vi "Generate Simulated Data.vi"(6 "Acquisition":refnum<queue>, 8 "error in (no error)":errorcluster, 10 "Longueur d'onde":dbl, 11 "Loop Count":dbl) -> (0 "error out":errorcluster, 2 "Data Out":variant[](array[variant]), 3 "Disconnected":bool=TRUE)   [LabVIEW 2018, in "Acquisition.lvlib"]
doc: "Generates sample waveforms according to the signal type in the HW Config input."
uses:
  Acquisition.lvlib
  <vilib>/Analysis/NI_AALBase.lvlib
  GlobalVariable/GlobalPowerByTime.vi
  GlobalVariable/Globalt0.vi
  support/Message Queue/Message Queue.lvlib
  <vilib>/gmath/NI_Gmath.lvlib
  GlobalVariable/GlobalSet0.vi
  <vilib>/Analysis/NI_AALPro.lvlib
  GlobalVariable/GlobalPosXbyTime.vi
  GlobalVariable/GlobalPosYbyTime.vi
  GlobalVariable/GlobalProfileByTime.vi
  GlobalVariable/GlobalTimeStep.vi
  GlobalVariable/GlobalTensionByTime.vi
  GlobalVariable/GlobalTemperatureByTime.vi
  support/Message Queue/Enqueue Message (Single).vi
  <vilib>/gmath/interp.llb/Create Mesh Grid (2D) (x,y arrays).vi
  <vilib>/Analysis/2dsp.llb/2D Convolution (DBL).vi
  <vilib>/Analysis/baseanly.llb/Mean (DBL).vi
  <vilib>/DAQmx/create/channels.llb/DAQmx Create Channel (DO-Digital Output).vi
  <resource>/objmgr/daqmx.rc
  <vilib>/DAQmx/write.llb/DAQmx Write (Digital 1D Bool NChan 1Samp 1Line).vi
  <vilib>/DAQmx/create/channels.llb/DAQmx Create Channel (AI-Voltage-Basic).vi
  <vilib>/DAQmx/configure/timing.llb/DAQmx Timing (Sample Clock).vi
  <vilib>/DAQmx/read.llb/DAQmx Read (Analog 1D Wfm NChan NSamp).vi
  support/Message Queue/Message Cluster.ctl
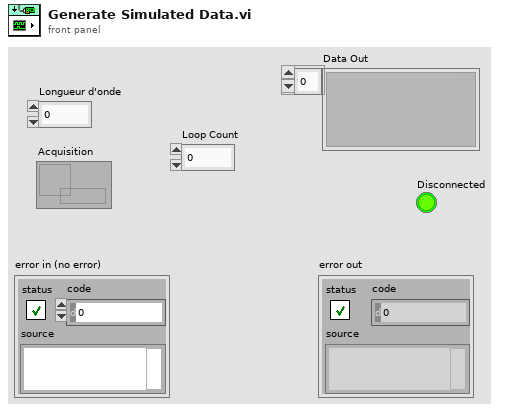
[diagram p1: front panel]
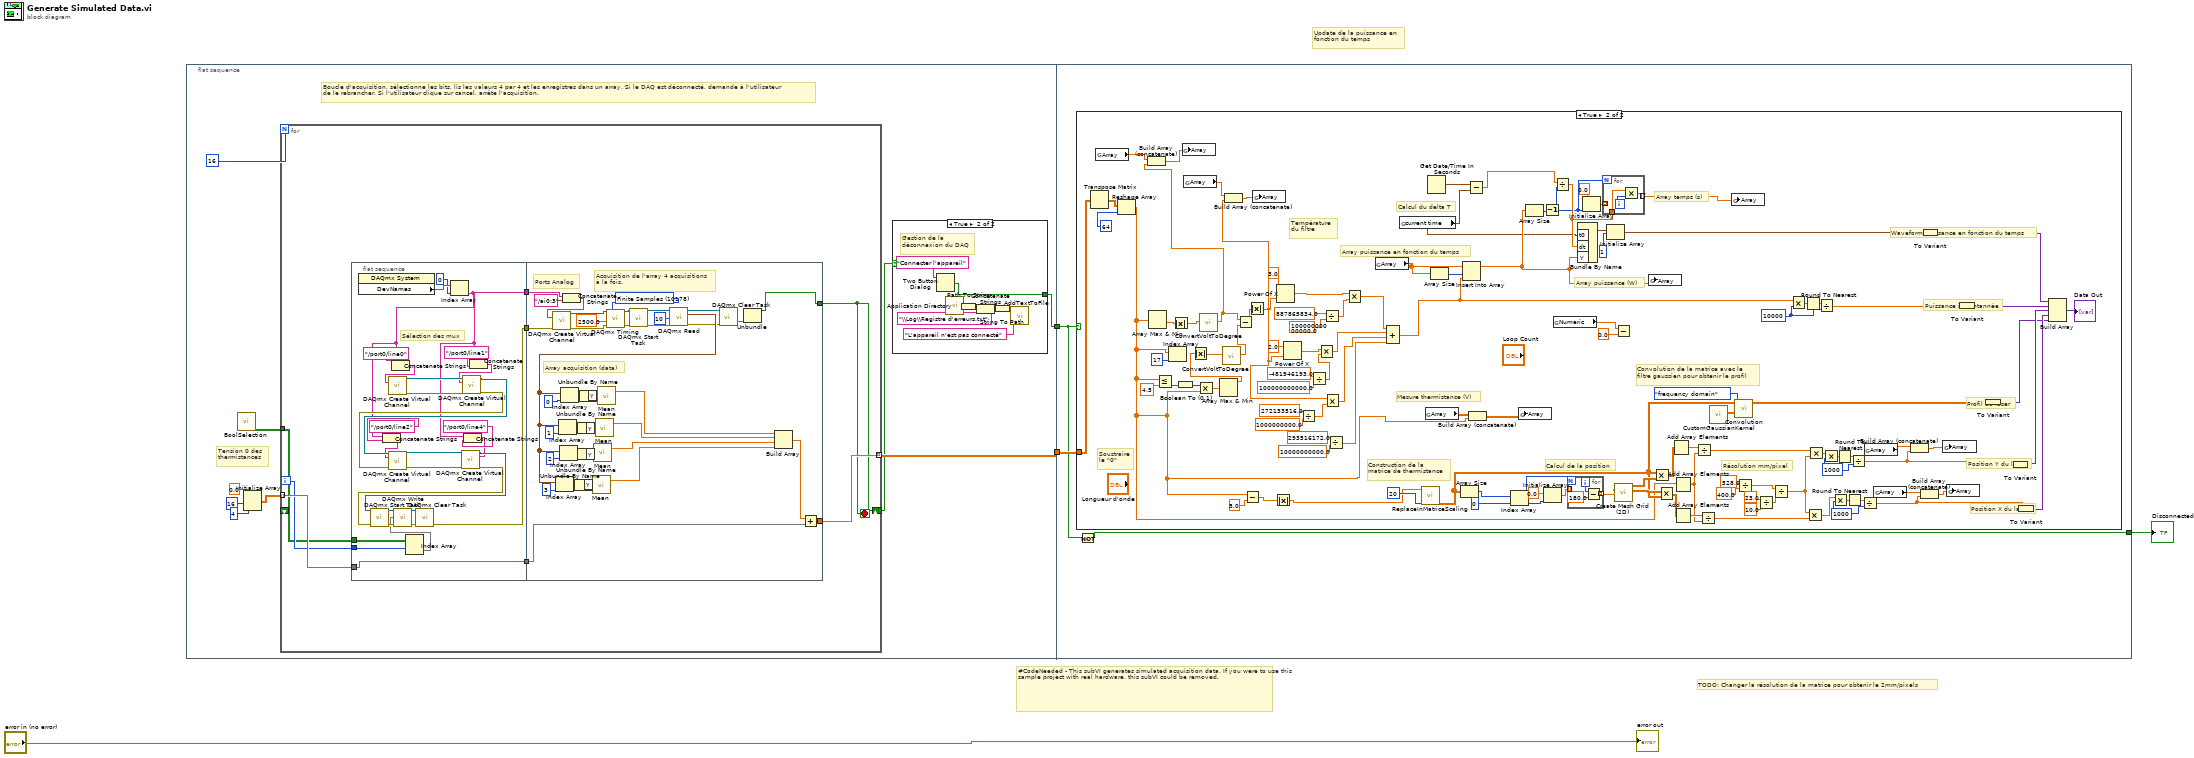
[diagram p0: block diagram]
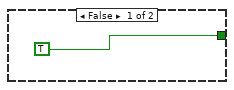
[diagram p2: hidden frame]
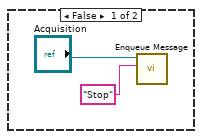
[diagram p3: hidden frame]
diagram:
  # "TODO: Changer la résolution de la matrice pour obtenir le 2mm/pixels"
  # "Update de la puissance en\nfonction du temps"
  # "#CodeNeeded - This subVI generates simulated acquisition data. If you were to use this sample project with real hardware, this subVI could be removed."
  n1 = flat-sequence {
    tunnel: [w11] -> w3
    tunnel: [w10] -> w2
    tunnel: w3 -> [w98]
    tunnel: w2 -> [w97]
    tunnel: [w96] -> w1
    frame #0 {
      # "Boucle d'acquisition, sélectionne les bits, lis les valeurs 4 par 4 et les enregistres dans un array. Si le DAQ est déconnecté, demande à l'utilisateur \nde le rebrancher. Si l'utilisateur clique sur cancel, arrête l'acquisition."
      # "Tension 0 des \nthermistances"
      n2 = call "BoolSelection.vi"() -> ("BoolSelection"=w12:bool[][])  [unwired: 11 in]
      n3 = Initialize Array(0.0 ("element"), 16 ("dimension size"), 4 ("dimension size")) -> (w6:dbl[][])
      n4 = for {
        N: 16 -> [_]
        tunnel: w12 -> [w25]
        tunnel: w6 -> [w30] mode=indexing
        tunnel: [w24] -> w11 mode=indexing
        shift-right: [w23] -> w5
        shift-left: _ -> [_]
        i -> [w26]
        stop <- w23 stop-if-true
        n5 = flat-sequence {
          tunnel: w26 -> [w44]
          tunnel: [w55] -> w29
          tunnel: w25 -> [w43]
          tunnel: [w31] -> w28
          tunnel: [w32] -> w27
          tunnel: w30 -> [w31]
          tunnel: w29 -> [w87]
          tunnel: w28 -> [w67]
          tunnel: [w69] -> w24
          tunnel: w27 -> [w64]
          tunnel: [w59] -> w23
          frame #0 {
            # "Sélection des mux"
            n6 = property class="DAQmx System"() -> ("DevNames"=w42:tag[])  [unwired: 2 in, 2 out]
            n7 = Index Array(array=w43, index (row)=w44) -> (element=w56:bool[])  [unwired: 1 in]
            n8 = Index Array(array=w42, index=0) -> (element=w32:tag)
            n9 = Concatenate Strings(w32, "/port0/line2" ("string")) -> (w35:string)
            n10 = Concatenate Strings(w32, "/port0/line0" ("string")) -> (w40:string)
            n11 = call-poly <vilib>:"DAQmx Create Virtual Channel.vi"("lines"=w40) -> ("task out"=w51:refnum<k21>, "error out"=w52:errorcluster)  [unwired: 13 in]
            n12 = Concatenate Strings(w32, "/port0/line4" ("string")) -> (w33:string)
            n13 = Concatenate Strings(w32, "/port0/line1" ("string")) -> (w37:string)
            n14 = call-poly <vilib>:"DAQmx Create Virtual Channel.vi"("task in"=w51, "lines"=w37, "error in"=w52) -> ("task out"=w50:refnum<k21>, "error out"=w49:errorcluster)  [unwired: 11 in]
            n15 = call-poly <vilib>:"DAQmx Create Virtual Channel.vi"("task in"=w50, "lines"=w35, "error in"=w49) -> ("task out"=w47:refnum<k21>, "error out"=w48:errorcluster)  [unwired: 11 in]
            n16 = call-poly <vilib>:"DAQmx Create Virtual Channel.vi"("task in"=w47, "lines"=w33, "error in"=w48) -> ("task out"=w46:refnum<k21>, "error out"=w45:errorcluster)  [unwired: 11 in]
            n17 = call <vilib>:"DAQmx Start Task.vi"("task/channels in"=w46, "error in"=w45) -> ("task out"=w57:refnum<k21>, "error out"=w58:errorcluster)  [unwired: 12 in]
            n18 = call-poly <vilib>:"DAQmx Write.vi"("task/channels in"=w57, "data"=w56, "error in"=w58) -> ("task out"=w54:refnum<k21>, "error out"=w53:errorcluster)  [unwired: 10 in, 1 out]
            n19 = call <vilib>:"DAQmx Clear Task.vi"("task in"=w54, "error in"=w53) -> ("error out"=w55:errorcluster)  [unwired: 13 in]
          }
          frame #1 {
            w89 = 10178 items=["Finite Samples"=10178, "Continuous Samples"=10123, "Hardware Timed Single Point"=12522] ("sample mode")
            # "Ports Analog"
            # "Array acquisition (data)"
            # "Acquisition de l'array 4 acquisitions\nà la fois."
            n20 = Concatenate Strings(w64, "/ai0:3" ("string")) -> (w65:string)
            n21 = call-poly <vilib>:"DAQmx Create Virtual Channel.vi"("physical channels"=w65, "error in"=w87) -> ("task out"=w94:refnum<k21>, "error out"=w93:errorcluster)  [unwired: 12 in]
            n22 = call-poly <vilib>:"DAQmx Timing.vi"("task/channels in"=w94, "sample mode"=w89, "rate"=2500.0, "error in"=w93) -> ("task out"=w90:refnum<k21>, "error out"=w91:errorcluster)  [unwired: 10 in]
            n23 = call <vilib>:"DAQmx Start Task.vi"("task/channels in"=w90, "error in"=w91) -> ("task out"=w92:refnum<k21>, "error out"=w95:errorcluster)  [unwired: 12 in]
            n24 = call-poly <vilib>:"DAQmx Read.vi"("task/channels in"=w92, "number of samples per channel"=10, "error in"=w95) -> ("task out"=w71:refnum<k21>, "data"=w80:waveform(dbl)[], "error out"=w70:errorcluster)  [unwired: 10 in]
            n25 = Index Array(array=w80, index=3) -> (element=w76:waveform(dbl))
            n26 = Index Array(array=w80, index=1) -> (element=w78:waveform(dbl))
            n27 = Index Array(array=w80, index=2) -> (element=w77:waveform(dbl))
            n28 = Index Array(array=w80, index=0) -> (element=w79:waveform(dbl))
            n29 = Unbundle By Name(w76) -> ("Y"=w72:dbl[])
            n30 = Unbundle By Name(w78) -> ("Y"=w74:dbl[])
            n31 = Unbundle By Name(w77) -> ("Y"=w73:dbl[])
            n32 = Unbundle By Name(w79) -> ("Y"=w75:dbl[])
            n33 = call-poly <vilib>:"Mean.vi"("X"=w72) -> ("mean"=w60:dbl)  [unwired: 1 out]
            n34 = call-poly <vilib>:"Mean.vi"("X"=w73) -> ("mean"=w61:dbl)  [unwired: 1 out]
            n35 = call-poly <vilib>:"Mean.vi"("X"=w74) -> ("mean"=w62:dbl)  [unwired: 1 out]
            n36 = call-poly <vilib>:"Mean.vi"("X"=w75) -> ("mean"=w63:dbl)  [unwired: 1 out]
            n37 = call <vilib>:"DAQmx Clear Task.vi"("task in"=w71, "error in"=w70) -> ("error out"=w85:errorcluster)  [unwired: 13 in]
            n38 = Unbundle(w85) -> ("status"=w59:bool)  [unwired: 2 out]
            n39 = Build Array(w63, w62, w61, w60) -> (w68:dbl[])
            n40 = Add(x=w68, y=w67) -> (x+y=w69:dbl[])
          }
        }
      }
      n41 = case shown="True" w5 {
        tunnel: [TRUE w22] -> w10
        frame False {
        }
        frame True {
          # "Gestion de la \ndéconnexion du DAQ"
          n42 = Two Button Dialog(message="Connecter l'appareil") -> (T button?=w22:bool)  [unwired: 2 in]
          n43 = call <vilib>:"Application Directory.vi"() -> ("Application Directory"=w19:path)
          n44 = Path To String(path=w19) -> (string=w20:string)
          n45 = Concatenate Strings(w20, "\\Log\\Registre d'erreurs.txt") -> (w21:string)
          n46 = String To Path(string=w21) -> (path=w17:path)
          n47 = call "AddTextToFile.vi"("Ajouter du texte"="L'appareil n'est pas connecté", "Fichier"=w17) -> ()  [unwired: 10 in]
        }
      }
    }
    frame #1 {
      n48 = case shown="True" w97 {
        tunnel: w98 -> [_ w167]
        frame False {
          n49 = call-poly "Enqueue Message.vi"("Message"="Stop", "Message Queue"="Acquisition") -> ()  [unwired: 8 in, 2 out]
        }
        frame True {
          w174 = 1000
          w178 = 1000
          w184 = 10000
          # "Résolution mm/pixel"
          # "Calcul du delta T"
          # "Mesure thermistance (V)"
          # "Soustraire\nle \"0\""
          # "Température \ndu filtre"
          # "Calcul de la position"
          # "Construction de la \nmatrice de thermistance"
          # "Position X du laser"
          # "Position Y du laser"
          # "Profil du laser"
          # "Puissance instantannée"
          # "Waveform puissance en fonction du temps"
          # "Array puissance (W)"
          # "Array temps (s)"
          # "Convolution de la matrice avec le \nfiltre gaussien pour obtenir le profil"
          # "Array puissance en fonction du temps"
          n50 = Transpose Matrix(1:w167) -> (0:w168:dbl[][])
          n51 = global read "GlobalTensionByTime.vi" "Array"() -> (w151:dbl[])
          n52 = Reshape Array(w168, 64 ("dimension size")) -> (w102:dbl[])
          n53 = Array Max & Min(array=w102) -> (min value=w118:dbl)  [unwired: 3 out]
          n54 = Less Or Equal?(x=w102, y=4.5) -> (x <= y?=w106:bool[])
          n55 = Index Array(array=w102, index=17) -> ()  [unwired: 1 out]
          n56 = Absolute Value(x=w118) -> (abs(x)=w112:dbl)
          n57 = Boolean To (0,1)(Boolean=w106) -> (0, 1=w105:i16[])
          n58 = global read "GlobalTemperatureByTime.vi" "Array"() -> (w148:dbl[])
          n59 = Multiply(x=w105, y=w102) -> (x*y=w104:dbl[])
          n60 = call "ConvertVoltToDegree.vi"("Tension"=w112) -> ("Température"=w113:dbl)  [unwired: 10 in]
          n61 = Build Array (concatenate)(w151, w113) -> (w150:dbl[])
          n62 = global write "GlobalTensionByTime.vi" "Array"(w150) -> ()
          n63 = Array Max & Min(array=w104) -> (max value=w103:dbl)  [unwired: 3 out]
          n64 = Absolute Value(x=w103) -> (abs(x)=w116:dbl)
          n65 = call "ConvertVoltToDegree.vi"("Tension"=w116) -> ("Température"=w115:dbl)  [unwired: 10 in]
          n66 = Subtract(x=w113, y=w115) -> (x-y=w117:dbl)
          n67 = Subtract(x=w102, y=5.0) -> (x-y=w108:dbl[])
          n68 = Absolute Value(x=w117) -> (abs(x)=w114:dbl)
          n69 = Build Array (concatenate)(w148, w114) -> (w149:dbl[])
          n70 = global write "GlobalTemperatureByTime.vi" "Array"(w149) -> ()
          n71 = Absolute Value(x=w108) -> (abs(x)=w101:dbl[])
          n72 = Power Of X(1:w114, 2:3.0 ("y")) -> (0:w122:dbl)
          n73 = Power Of X(1:w114, 2:2.0 ("y")) -> (0:w134:dbl)
          n74 = Divide(x=272133516.0, y=1000000000.0) -> (x/y=w130:dbl)
          n75 = Divide(x=-481946193.0, y=100000000000.0) -> (x/y=w133:dbl)
          n76 = Multiply(x=w134, y=w133) -> (x*y=w123:dbl)
          n77 = Divide(x=887865834.0, y=10000000000000.0) -> (x/y=w121:dbl)
          n78 = Multiply(x=w114, y=w130) -> (x*y=w124:dbl)
          n79 = Divide(x=293516172.0, y=10000000000.0) -> (x/y=w125:dbl)
          n80 = Multiply(x=w122, y=w121) -> (x*y=w120:dbl)
          n81 = global read "GlobalPowerByTime.vi" "Array"() -> (w214:dbl[])
          n82 = Compound Arithmetic op=ADD(w120, w123, w124, w125) -> (w126:dbl)
          n83 = global read "Globalt0.vi" "current time"() -> (w153:timestamp)
          n84 = call "ReplaceInMatriceScaling.vi"("Input Scaling"=20, "Input Array"=w101) -> ("Output Array"=w110:dbl[][])  [unwired: 9 in]
          n85 = global read "GlobalProfileByTime.vi" "Array"() -> (w157:dbl[][])
          n86 = Get Date/Time In Seconds() -> (seconds since 1Jan1904=w154:timestamp)
          n87 = Array Size(array=w214) -> (size(s)=w213:i32)
          n88 = Array Size(array=w110) -> (size(s)=w205:i32[])
          n89 = Insert Into Array(array=w214, index=w213, new element=w126) -> (w166:dbl[])
          n90 = Subtract(x=w154, y=w153) -> (x-y=w152:dbl)
          n91 = Build Array (concatenate)(w157, w102) -> (w158:dbl[][])
          n92 = Index Array(array=w205, index=0) -> (element=w200:i32)
          n93 = global write "GlobalProfileByTime.vi" "Array"(w158) -> ()
          n94 = Array Size(array=w166) -> (size(s)=w156:i32)
          n95 = Decrement(x=w156) -> (x-1=w155:i32)
          n96 = Initialize Array(0.0 ("element"), w200) -> (w202:dbl[])
          n97 = global read "GlobalSet0.vi" "Numeric"() -> (w141:dbl)
          n98 = Divide(x=w152, y=w155) -> (x/y=w209:dbl)
          n99 = for {
            N: w200 -> [_]
            tunnel: w202 -> [_] mode=indexing
            tunnel: [w215] -> w197 mode=indexing
            i -> [w216]
            n100 = Subtract(x=w216, y=180.0) -> (x-y=w215:dbl)
          }
          n101 = Bundle By Name("t0"=w153, "dt"=w209, "Y"=w166) -> (w211:waveform(dbl))  [unwired: 1 in]
          n102 = Initialize Array(0.0 ("element"), w155) -> (w207:dbl[])
          n103 = for {
            N: w155 -> [_]
            tunnel: w209 -> [w219]
            tunnel: w207 -> [_] mode=indexing
            tunnel: [w218] -> w165 mode=indexing
            i -> [w220]
            n104 = Multiply(x=w219, y=w220) -> (x*y=w218:dbl)
          }
          n105 = Initialize Array(w211, 1) -> (w188:waveform(dbl)[])
          n106 = call-poly <vilib>:"Create Mesh Grid (2D).vi"("y domain"=w197, "x domain"=w197) -> ("Y"=w196:dbl[][], "X"=w201:dbl[][])  [unwired: 7 in, 1 out]
          n107 = Subtract(x=w141, y=0.0) -> ()  [unwired: 1 out]
          n108 = global write "GlobalPowerByTime.vi" "Array"(w166) -> ()
          n109 = Multiply(x=w110, y=w201) -> (x*y=w199:dbl[][])
          n110 = Multiply(x=w196, y=w110) -> (x*y=w195:dbl[][])
          n111 = Add Array Elements(numeric array=w199) -> (sum=w198:dbl)
          n112 = Add Array Elements(numeric array=w102) -> (sum=w193:dbl)
          n113 = Add Array Elements(numeric array=w195) -> (sum=w194:dbl)
          n114 = Divide(x=w198, y=w193) -> (x/y=w191:dbl)
          n115 = Divide(x=w194, y=w193) -> (x/y=w192:dbl)
          n116 = call "CustomGaussianKernel.vi"() -> ("array"=w206:dbl[][])  [unwired: 11 in]
          n117 = global write "GlobalTimeStep.vi" "Array"(w165) -> ()
          n118 = call-poly <vilib>:"Convolution.vi"("algorithm"=enum32{"direct", "frequency domain"}."frequency domain", "Y"=w206, "X"=w110) -> ("X * Y"=w142:dbl[][])  [unwired: 7 in, 1 out]
          n119 = Divide(x=528.0, y=400.0) -> (x/y=w145:dbl)
          n120 = Divide(x=23.0 ("y"), y=10.0) -> (x/y=w144:dbl)
          n121 = Divide(x=w145, y=w144) -> (x/y=w143:dbl)
          n122 = Multiply(x=w126, y=w184) -> (x*y=w185:dbl)
          n123 = Round To Nearest(number=w185) -> (nearest integer value=w183:dbl)
          n124 = Multiply(x=w143, y=w192) -> (x*y=w171:dbl)
          n125 = Multiply(x=w191, y=w143) -> (x*y=w175:dbl)
          n126 = Divide(x=w183, y=w184) -> (x/y=w179:dbl)
          n127 = Multiply(x=w175, y=w178) -> (x*y=w177:dbl)
          n128 = Multiply(x=w171, y=w174) -> (x*y=w173:dbl)
          n129 = Round To Nearest(number=w177) -> (nearest integer value=w176:dbl)
          n130 = Round To Nearest(number=w173) -> (nearest integer value=w172:dbl)
          n131 = Divide(x=w176, y=w178) -> (x/y=w159:dbl)
          n132 = Divide(x=w172, y=w174) -> (x/y=w163:dbl)
          n133 = global read "GlobalPosXbyTime.vi" "Array"() -> (w160:dbl[])
          n134 = global read "GlobalPosYbyTime.vi" "Array"() -> (w164:dbl[])
          n135 = Build Array (concatenate)(w160, w159) -> (w161:dbl[])
          n136 = Build Array (concatenate)(w164, w163) -> (w162:dbl[])
          n137 = To Variant(anything=w188) -> (Variant=w187:variant)
          n138 = global write "GlobalPosXbyTime.vi" "Array"(w161) -> ()
          n139 = global write "GlobalPosYbyTime.vi" "Array"(w162) -> ()
          n140 = To Variant(anything=w179) -> (Variant=w180:variant)
          n141 = To Variant(anything=w142) -> (Variant=w170:variant)
          n142 = To Variant(anything=w159) -> (Variant=w181:variant)
          n143 = To Variant(anything=w163) -> (Variant=w182:variant)
          n144 = Build Array(w187, w180, w181, w182, w170) -> (→"Data Out":variant[])
        }
      }
      n145 = Not(x=w97) -> (.not. x?=w96:bool)
    }
  }
  "error out" <- "error in (no error)"
  "Disconnected" <- w1
